vi "DeleteFromReservedList.vi"(11 "VISA resource":string) -> (3 "VISA resource out":string)   [LabVIEW 2019]
uses:
  GLOBALS.vi
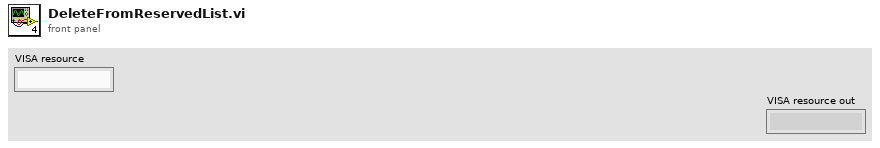
[diagram p1: front panel]
types:
  T1 = typedef "Globals_IO.ctl" = cluster{"Reserved COM ports":cluster{"Port":string, "Reserved By":string, "Time":timestamp}[]}
  T2 = cluster{"Port":string, "Reserved By":string, "Time":timestamp}[]
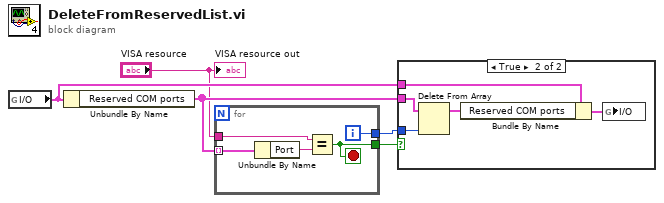
[diagram p0: block diagram]
diagram:
  n1 = global read "Globals.vi" "I/O"() -> (w3:T1)
  n2 = Unbundle By Name(w3) -> ("Reserved COM ports"=w2:T2)
  n3 = for {
    tunnel: [w9] -> w5
    tunnel: [w10] -> w4
    tunnel: w2 -> [w7] mode=indexing
    tunnel: "VISA resource" -> [w8]
    i -> [w10]
    stop <- w9 stop-if-true
    n4 = Unbundle By Name(w7) -> ("Port"=w6:string)
    n5 = Equal?(x=w8, y=w6) -> (x = y?=w9:bool)
  }
  n6 = case shown="True" w5 {
    tunnel: w4 -> [_ w12]
    tunnel: w3 -> [_ w15]
    tunnel: w2 -> [_ w13]
    frame False {
    }
    frame True {
      n7 = Delete From Array(array=w13, index=w12) -> (array with subset deleted=w11:T2)  [unwired: 1 in, 1 out]
      n8 = Bundle By Name(cluster=w15, "Reserved COM ports"=w11) -> (w14:T1)
      n9 = global write "Globals.vi" "I/O"(w14) -> ()
    }
  }
  "VISA resource out" <- "VISA resource"
